vi "unpack_extended_depth.vi"(10 "payload_size":u32, 11 "payload":u64) -> (0 "height":u16, 1 "width":u16, 2 "metadata":cluster{"width":u16, "height":u16}, 3 "image":u16[][](array[numeric]), 4 "error":bool)   [LabVIEW 2023]
panel:
  in  "extended_depth_metadata":cluster{"width":u16, "height":u16}
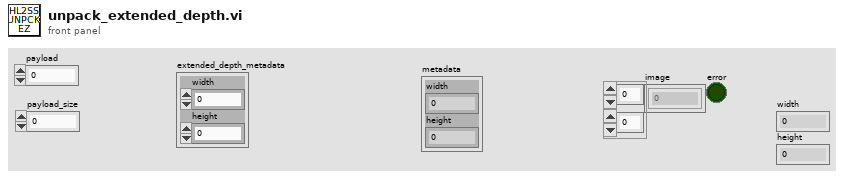
[diagram p1: front panel]
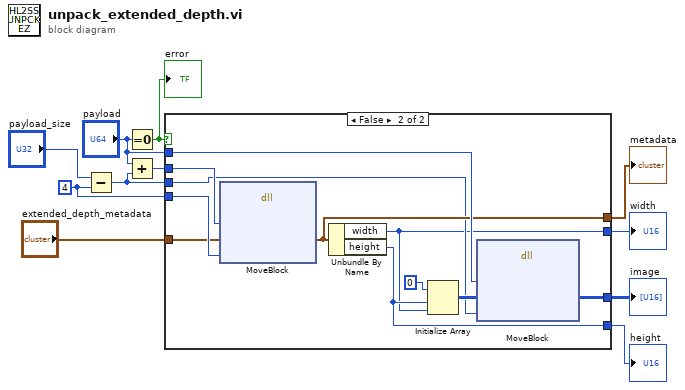
[diagram p0: block diagram]
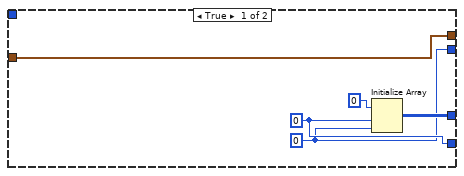
[diagram p2: hidden frame]
diagram:
  w6 = u64 4 ("size")
  n1 = Subtract(x="payload_size", y=w6) -> (x-y=w4:u64)
  n2 = Equal To 0?(x="payload") -> (x = 0?=w7:bool)
  "error" <- w7
  n3 = Add(x="payload", y=w4) -> (x+y=w11:u64)
  n4 = case shown="False" w7 {
    tunnel: "payload" -> [_ w27]
    tunnel: w11 -> [_ w26]
    tunnel: w6 -> [_ w25]
    tunnel: "extended_depth_metadata" -> [w16 w24]
    tunnel: [w16 w21] -> w9
    tunnel: w4 -> [_ w20]
    tunnel: [w14 w19] -> w3
    tunnel: [w13 w18] -> w2
    tunnel: [w12 w17] -> w1
    frame True {
      w12 = u16 0 ("dimension size")
      w13 = u16 0 ("dimension size")
      n5 = Initialize Array(u16 0, w13, w12) -> (w14:u16[][])
    }
    frame False {
      n6 = dll-call lib="LabVIEW" fn="MoveBlock"("ps"=w26, "pd"=w24, "size"=w25) -> ("pd"=w21:cluster{"width":u16, "height":u16})  [unwired: 6 in, 2 out]
      n7 = Unbundle By Name(w21) -> ("width"=w17:u16, "height"=w18:u16)
      n8 = Initialize Array(u16 0, w18, w17) -> (w22:u16[][])
      n9 = dll-call lib="LabVIEW" fn="MoveBlock"("ps"=w27, "pd"=w22, "size"=w20) -> ("pd"=w19:u16[][])  [unwired: 6 in, 2 out]
    }
  }
  "image" <- w3
  "metadata" <- w9
  "width" <- w1
  "height" <- w2
